vi "LVIS_CalcTestResult.vi"(8 "Error In":errorcluster, 11 "MeasStatus":string) -> (0 "Error out":errorcluster, 3 "TestInfo":T1)   [LabVIEW 2015]
doc: "Determines the test status based on relevent measurement status."
uses:
  Globals/LVIS_IsGlobal.vi
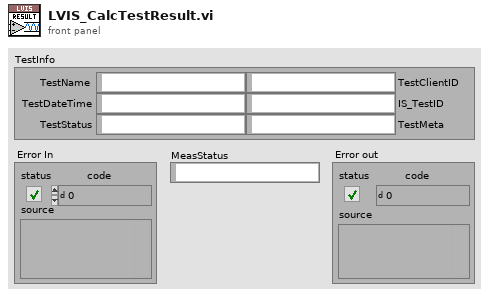
[diagram p1: front panel]
types:
  T1 = cluster{"TestName":string, "TestDateTime":string, "TestStatus":string, "TestClientID":string, "IS_TestID":string, "TestMeta":string}
  T2 = cluster{"EventInfo":cluster{"EventName":string, "EventStart":string, "EventStop":string, "EventStatus":string, "EventClientID":string, "IS_EventID":string, "EventMeta":string, "ProductLine":string, "ProcessName":string, "Station":string, "Operator":string, "SN":string, "Model":string, "Manufacturer":string}, "TestInfo":cluster{"TestName":string, "TestDateTime":string, "TestStatus":string, "TestClientID":string, "IS_TestID":string, "TestMeta":string}, "MeasInfo":cluster{"MeasName":string, "MeasDateTime":string, "MeasStatus":string, "MeasClientID":string, "IS_MeasID":string, "MeasMeta":string, "MeasType":string, "MeasValue":string, "LL":string, "LL Comp":string, "HL":string, "HL Comp":string, "Units":string}}[]
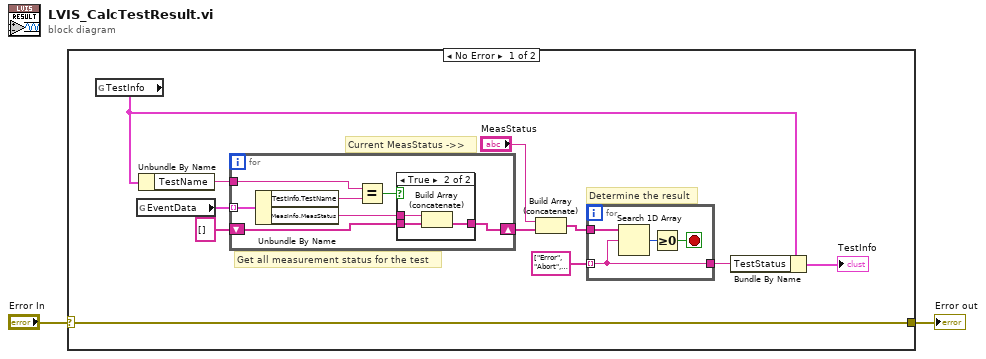
[diagram p0: block diagram]
diagram:
  n1 = case shown="No Error" "Error In" {
    selector: "Error In" -> [w13 w29]
    tunnel: [w13 w29] -> w1
    frame No Error {
      # "Current MeasStatus ->>"
      # "Determine the result"
      # "Get all measurement status for the test"
      n2 = global read "LVIS_IsGlobal.vi" "TestInfo"() -> (w3:T1)
      n3 = global read "LVIS_IsGlobal.vi" "EventData"() -> (w12:T2)
      n4 = Unbundle By Name(w3) -> ("TestName"=w11:string)
      n5 = for {
        tunnel: w12 -> [w24] mode=indexing
        tunnel: w11 -> [w22]
        shift-right: [w18] -> w5
        shift-left: string[] [] -> [w19]
        n6 = Unbundle By Name(w24) -> ("TestInfo.TestName"=w23:string, "MeasInfo.MeasStatus"=w20:string)
        n7 = Equal?(x=w22, y=w23) -> (x = y?=w21:bool)
        n8 = case shown="True" w21 {
          tunnel: w20 -> [_ w28]
          tunnel: w19 -> [w25 w27]
          tunnel: [w25 w26] -> w18
          frame False {
          }
          frame True {
            n9 = Build Array (concatenate)(w28, w27) -> (w26:string[])
          }
        }
      }
      n10 = Build Array (concatenate)("MeasStatus", w5) -> (w6:string[])
      n11 = for {
        tunnel: w6 -> [w17]
        tunnel: string[] ["Error", "Abort", "Failed", "Passed", "Logged"] -> [w15] mode=indexing
        tunnel: [w15] -> w8
        stop <- w14 stop-if-true
        n12 = Search 1D Array(1D array=w17, element=w15) -> (index of element=w16:i32)  [unwired: 1 in]
        n13 = Greater Or Equal To 0?(x=w16) -> (x >= 0?=w14:bool)
      }
      n14 = Bundle By Name(cluster=w3, "TestStatus"=w8) -> (→"TestInfo":T1)
    }
    frame Error {
    }
  }
  "Error out" <- w1
